vi "Read Config.vi"(8 "error in (no error)":errorcluster) -> (0 "error out":errorcluster, 1 "Serial No_KIA":string, 2 "Configuration":refnum<vi>, 3 "Configuration Read":T1={"Model"=enum."KIA", "Shift A From"={"Hour"=0, "  Minutes"=0}, "Shift A To"={"Hour"=0, "  Minutes"=0}, "Shift B From"={"Hour"=0, "  Minutes"=0}, "Shift B To"={"Hour"=0, "  Minutes"=0}, "Shift C From"={"Hour"=0, "  Minutes"=0}, "Shift C To"={"Hour"=0, "  Minutes"=0}, "Shifts"=enum."Shift A", "Device Configurations"={"PLC Configurations"={"PLC IP"="", "Port"=102, "Datablock"=102}, "TG Configuration"={"IP Adress"="", "Port"=0}, "Printer Configuration"={"IP Adress"="", "Port"=0}, "Scanner Configuration"={"IP Adress"="", "Port"=0}}, "Report File Path"=path "", "Reprint Label"=FALSE} {"Shift C From"."Minutes" items=["00", "01", "02", "03", "04", "05", "06", "07", "08", "09", "10", "11", "12", "13", "14", "15", "16", "17", "18", "19", "20", "21", "22", "23", "24", "25", "26", "27", "28", "29", "30", "31", "32", "33", "34", "35", "36", "37", "38", "39", "40", "41", "42", "43", "44", "45", "46", "47", "48", "49", "50", "51", "52", "53", "54", "55", "56", "57", "58", "59"]; "Shift C From"."Hour" items=["00", "01", "02", "03", "04", "05", "06", "07", "08", "09", "10", "11", "12", "13", "14", "15", "16", "17", "18", "19", "20", "21", "22", "23"]; "Shift C To"."Minutes" items=["00", "01", "02", "03", "04", "05", "06", "07", "08", "09", "10", "11", "12", "13", "14", "15", "16", "17", "18", "19", "20", "21", "22", "23", "24", "25", "26", "27", "28", "29", "30", "31", "32", "33", "34", "35", "36", "37", "38", "39", "40", "41", "42", "43", "44", "45", "46", "47", "48", "49", "50", "51", "52", "53", "54", "55", "56", "57", "58", "59"]; "Shift C To"."Hour" items=["00", "01", "02", "03", "04", "05", "06", "07", "08", "09", "10", "11", "12", "13", "14", "15", "16", "17", "18", "19", "20", "21", "22", "23"]; "Shift B To"."Minutes" items=["00", "01", "02", "03", "04", "05", "06", "07", "08", "09", "10", "11", "12", "13", "14", "15", "16", "17", "18", "19", "20", "21", "22", "23", "24", "25", "26", "27", "28", "29", "30", "31", "32", "33", "34", "35", "36", "37", "38", "39", "40", "41", "42", "43", "44", "45", "46", "47", "48", "49", "50", "51", "52", "53", "54", "55", "56", "57", "58", "59"]; "Shift B To"."Hour" items=["00", "01", "02", "03", "04", "05", "06", "07", "08", "09", "10", "11", "12", "13", "14", "15", "16", "17", "18", "19", "20", "21", "22", "23"]; "Shift B From"."Minutes" items=["00", "01", "02", "03", "04", "05", "06", "07", "08", "09", "10", "11", "12", "13", "14", "15", "16", "17", "18", "19", "20", "21", "22", "23", "24", "25", "26", "27", "28", "29", "30", "31", "32", "33", "34", "35", "36", "37", "38", "39", "40", "41", "42", "43", "44", "45", "46", "47", "48", "49", "50", "51", "52", "53", "54", "55", "56", "57", "58", "59"]; "Shift B From"."Hour" items=["00", "01", "02", "03", "04", "05", "06", "07", "08", "09", "10", "11", "12", "13", "14", "15", "16", "17", "18", "19", "20", "21", "22", "23"]; "Shift A To"."Minutes" items=["00", "01", "02", "03", "04", "05", "06", "07", "08", "09", "10", "11", "12", "13", "14", "15", "16", "17", "18", "19", "20", "21", "22", "23", "24", "25", "26", "27", "28", "29", "30", "31", "32", "33", "34", "35", "36", "37", "38", "39", "40", "41", "42", "43", "44", "45", "46", "47", "48", "49", "50", "51", "52", "53", "54", "55", "56", "57", "58", "59"]; "Shift A To"."Hour" items=["00", "01", "02", "03", "04", "05", "06", "07", "08", "09", "10", "11", "12", "13", "14", "15", "16", "17", "18", "19", "20", "21", "22", "23"]; "Shift A From"."Minutes" items=["00", "01", "02", "03", "04", "05", "06", "07", "08", "09", "10", "11", "12", "13", "14", "15", "16", "17", "18", "19", "20", "21", "22", "23", "24", "25", "26", "27", "28", "29", "30", "31", "32", "33", "34", "35", "36", "37", "38", "39", "40", "41", "42", "43", "44", "45", "46", "47", "48", "49", "50", "51", "52", "53", "54", "55", "56", "57", "58", "59"]; "Shift A From"."Hour" items=["00", "01", "02", "03", "04", "05", "06", "07", "08", "09", "10", "11", "12", "13", "14", "15", "16", "17", "18", "19", "20", "21", "22", "23"]})   [LabVIEW 2021]
uses:
  <vilib>/Utility/config.llb/NI_LVConfig.lvlib
  Gen fgv action.ctl
  C/Users/enProducts/Downloads/KIA_Enproducts/KIA_Enproducts/Configuration/Controls/Part Model.ctl
  C/Users/enProducts/Downloads/KIA_Enproducts/KIA_Enproducts/Configuration/Controls/Hour Control.ctl
  C/Users/enProducts/Downloads/KIA_Enproducts/KIA_Enproducts/Configuration/Controls/Minute Control.ctl
  C/Users/enProducts/Downloads/KIA_Enproducts/KIA_Enproducts/Device Manager/Device Config.ctl
  C/Users/enProducts/Downloads/KIA_Enproducts/KIA_Enproducts/Configuration/Controls/Configuration.ctl
  C/Users/enProducts/Downloads/KIA_Enproducts/KIA_Enproducts/Global VIs/Controls/Read Write.ctl
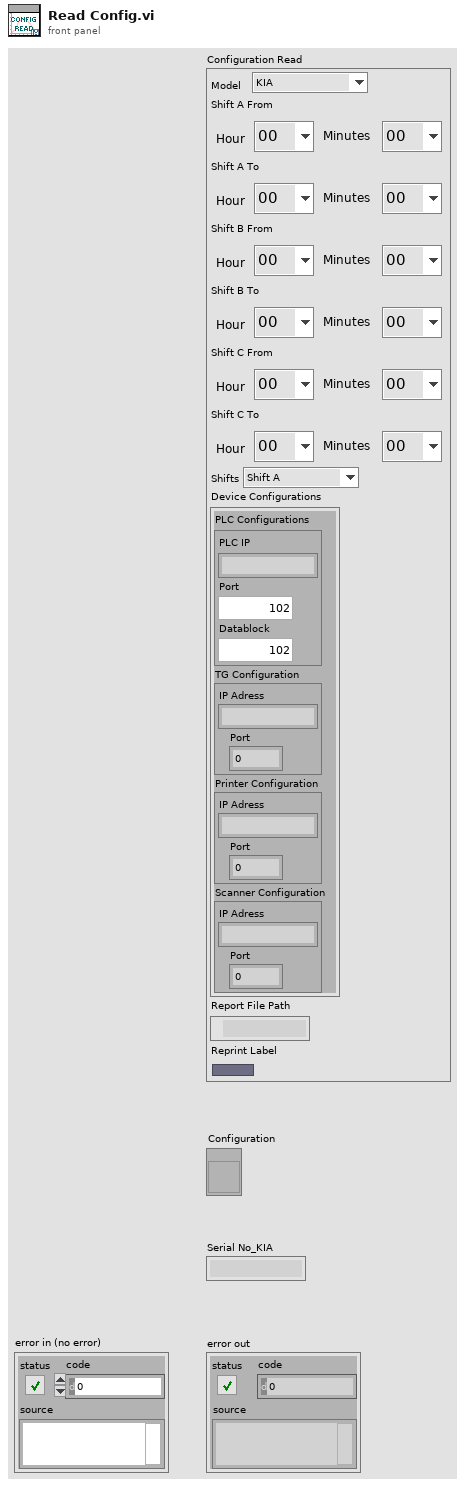
[diagram p1: front panel]
types:
  T1 = typedef "Configuration.ctl" = cluster{"Model":T2, "Shift A From":cluster{"Hour":T3, "  Minutes":T4}, "Shift A To":cluster{"Hour":T3, "  Minutes":T4}, "Shift B From":cluster{"Hour":T3, "  Minutes":T4}, "Shift B To":cluster{"Hour":T3, "  Minutes":T4}, "Shift C From":cluster{"Hour":T3, "  Minutes":T4}, "Shift C To":cluster{"Hour":T3, "  Minutes":T4}, "Shifts":enum16{"Shift A", "Shift B", "Shift C"}, "Device Configurations":T5, "Report File Path":path, "Reprint Label":bool}
  T2 = typedef "Part Model.ctl" = enum16{"KIA"}
  T3 = typedef "Hour Control.ctl" = u16
  T4 = typedef "Minute Control.ctl" = u16
  T5 = typedef "Device Config.ctl" = cluster{"PLC Configurations":cluster{"PLC IP":string, "Port":u16, "Datablock":u16}, "TG Configuration":cluster{"IP Adress":string, "Port":i16}, "Printer Configuration":cluster{"IP Adress":string, "Port":i16}, "Scanner Configuration":cluster{"IP Adress":string, "Port":i16}}
  T6 = typedef "Gen FGV Action.ctl" = enum16{"Initialize", "Get Data", "Update Data", "Clear Data"}
  T7 = typedef "Read Write.ctl" = enum16{"Read", "Write"}
  T8 = enum16{"open", "replace", "create", "open or create", "replace or create", "replace or create with confirmation"}
  T9 = typedef "File Paths.ctl" = cluster{"Log":path, "Report":path, "Error Info":path, "Event log":path, "Configuration":path, "Database":path, "Test Statistics":path, "User Accounts":path, "Video Folder":path, "Crimping Report":path}
  T10 = typedef "NI_LVConfig.lvlib/Config Data RefNum.ctl" = refnum<k1>
  T11 = typedef "SERIAL N0.ctl" = string
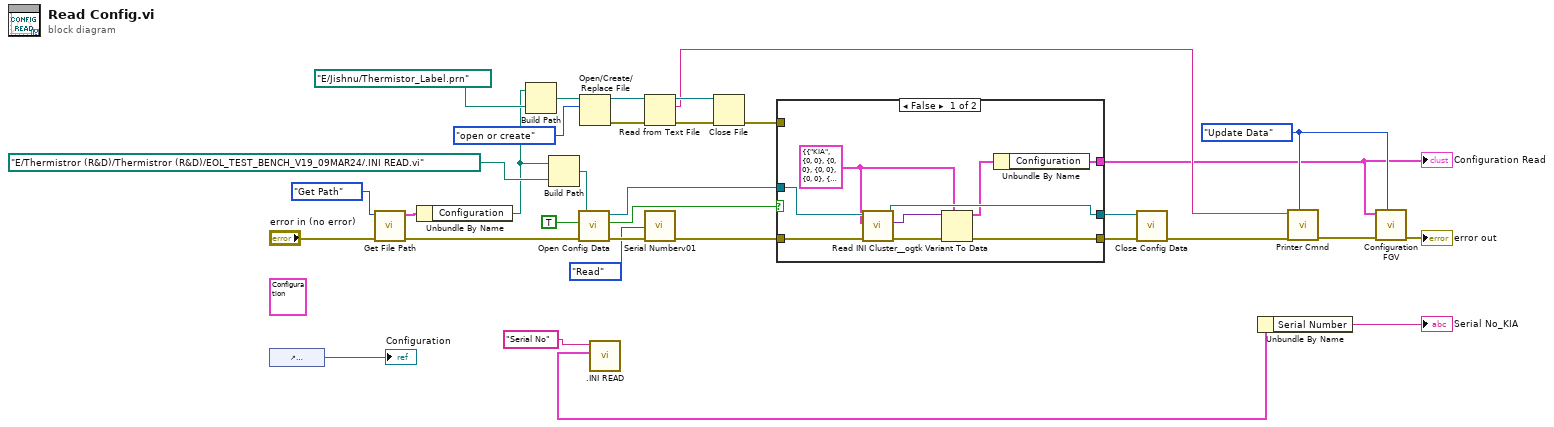
[diagram p0: block diagram]
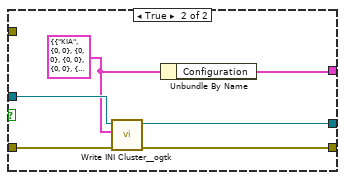
[diagram p2: hidden frame]
diagram:
  w9 = Gen_FGV_Action."Update Data" ("Action?")
  (unwired) T1 {"Model"=enum."KIA", "Shift A From"={"Hour"=0, "  Minutes"=0}, "Shift A To"={"Hour"=0, "  Minutes"=0}, "Shift B From"={"Hour"=0, "  Minutes"=0}, "Shift B To"={"Hour"=0, "  Minutes"=0}, "Shift C From"={"Hour"=0, "  Minutes"=0}, "Shift C To"={"Hour"=0, "  Minutes"=0}, "Shifts"=enum."Shift A", "Device Configurations"={"PLC Configurations"={"PLC IP"="", "Port"=102, "Datablock"=102}, "TG Configuration"={"IP Adress"="", "Port"=0}, "Printer Configuration"={"IP Adress"="", "Port"=0}, "Scanner Configuration"={"IP Adress"="", "Port"=0}}, "Report File Path"=path "", "Reprint Label"=FALSE} ("Configuration")
  n1 = control-ref of="Configuration Read"() -> (→"Configuration":refnum<vi>)
  n2 = call "Get File Path.vi"("error in (no error)"="error in (no error)", "Action?"=enum16{"Initialize", "Get Path"}."Get Path") -> ("error out"=w24:errorcluster, "File Paths"=w33:T9)  [unwired: 8 in]
  n3 = Unbundle By Name(w33) -> ("Configuration"=w19:path)
  n4 = Build Path(base path=w19, name or relative path=path "E:/Jishnu/Thermistor_Label.prn") -> (appended path=w21:path)
  n5 = Build Path(base path=w19, name or relative path=path "E:/Thermistror (R&D)/Thermistror (R&D)/EOL_TEST_BENCH_V19_09MAR24/.INI READ.vi") -> (appended path=w18:path)
  n6 = call <vilib>:"Open Config Data.vi"("error in (no error)"=w24, "create file if necessary (T)"=TRUE, "configuration file path"=w18) -> ("error out"=w14:errorcluster, "file created?"=w27:bool, "refnum"=w17:T10)  [unwired: 6 in]
  n7 = Open/Create/Replace File(file path (use dialog)=w21, operation (0:open)=T8."open or create") -> (refnum out=w20:refnum<file>, error out=w22:errorcluster)  [unwired: 4 in, 1 out]
  n8 = call ".INI READ.vi"("KEY"="Serial No") -> ("Serail No"=w2:cluster{"Serial Number":T11})  [unwired: 3 in, 7 out]
  n9 = Read from Text File(file (use dialog)=w20, error in=w22) -> (refnum out=w15:refnum<file>, text=w8:string, error out=w10:errorcluster)  [unwired: 2 in, 1 out]
  n10 = call "Serial Numberv01.vi"("error in"=w14, "Read Write"=Read_Write."Read") -> ("error out"=w13:errorcluster)  [unwired: 8 in, 1 out]
  n11 = Close File(refnum=w15, error in=w10) -> (error out=w7:errorcluster)  [unwired: 1 out]
  n12 = case shown="False" w27 {
    tunnel: w17 -> [w42 w47]
    tunnel: w13 -> [w39 w48]
    tunnel: [w41 w45] -> w26
    tunnel: [w38 w46] -> w25
    tunnel: [w35 w43] -> w3
    tunnel: w7 -> [_ _]
    frame False {
      w36 = cluster{"Configuration":T1} {"Configuration"={"Model"=enum."KIA", "Shift A From"={"Hour"=0, "  Minutes"=0}, "Shift A To"={"Hour"=0, "  Minutes"=0}, "Shift B From"={"Hour"=0, "  Minutes"=0}, "Shift B To"={"Hour"=0, "  Minutes"=0}, "Shift C From"={"Hour"=0, "  Minutes"=0}, "Shift C To"={"Hour"=0, "  Minutes"=0}, "Shifts"=enum."Shift A", "Device Configurations"={"PLC Configurations"={"PLC IP"="", "Port"=102, "Datablock"=102}, "TG Configuration"={"IP Adress"="", "Port"=0}, "Printer Configuration"={"IP Adress"="", "Port"=0}, "Scanner Configuration"={"IP Adress"="", "Port"=0}}, "Report File Path"=path "", "Reprint Label"=FALSE}}
      n13 = call <userlib>:"Read INI Cluster__ogtk.vi"("error in (no error)"=w39, "INI Fomatted Cluster Type"=w36, "refnum"=w42) -> ("error out"=w34:errorcluster, "INI Fomatted Cluster"=w40:variant, "dup refnum"=w41:T10)  [unwired: 4 in, 2 out]
      n14 = Variant To Data(error in=w34, type=w36, Variant=w40) -> (data=w37:cluster{"Configuration":T1}, error out=w38:errorcluster)
      n15 = Unbundle By Name(w37) -> ("Configuration"=w35:T1)
    }
    frame True {
      w44 = cluster{"Configuration":T1} {"Configuration"={"Model"=enum."KIA", "Shift A From"={"Hour"=0, "  Minutes"=0}, "Shift A To"={"Hour"=0, "  Minutes"=0}, "Shift B From"={"Hour"=0, "  Minutes"=0}, "Shift B To"={"Hour"=0, "  Minutes"=0}, "Shift C From"={"Hour"=0, "  Minutes"=0}, "Shift C To"={"Hour"=0, "  Minutes"=0}, "Shifts"=enum."Shift A", "Device Configurations"={"PLC Configurations"={"PLC IP"="", "Port"=102, "Datablock"=102}, "TG Configuration"={"IP Adress"="", "Port"=0}, "Printer Configuration"={"IP Adress"="", "Port"=0}, "Scanner Configuration"={"IP Adress"="", "Port"=0}}, "Report File Path"=path "", "Reprint Label"=FALSE}}
      n16 = call <userlib>:"Write INI Cluster__ogtk.vi"("error in (no error)"=w48, "INI Fomatted Cluster"=w44, "refnum"=w47) -> ("error out"=w46:errorcluster, "dup refnum"=w45:T10)  [unwired: 7 in]
      n17 = Unbundle By Name(w44) -> ("Configuration"=w43:T1)
    }
  }
  "Configuration Read" <- w3
  n18 = call <vilib>:"Close Config Data.vi"("error in (no error)"=w25, "refnum"=w26) -> ("error out"=w6:errorcluster)  [unwired: 8 in, 1 out]
  n19 = Unbundle By Name(w2) -> ("Serial Number"=→"Serial No_KIA":T11)
  n20 = call "Printer Cmnd.vi"("Action?"=w9, "error in (no error)"=w6, "String"=w8) -> ("error out"=w5:errorcluster)  [unwired: 7 in, 1 out]
  n21 = call "Configuration FGV.vi"("Action?"=w9, "error in (no error)"=w5, "Configuration"=w3) -> ("error out"=→"error out":errorcluster)  [unwired: 7 in, 1 out]
